vi "PCU_Connect.vi"(0 "GPIBBoard":i32, 1 "Address/ComPort":string, 2 "Communication":T1(ring), 3 "Terminator":enum32{"Cr", "Lf", "CrLf"}(ring), 4 "Portnumber":i32, 5 "error in":errorcluster, 6 "Target":enum32{"rdo100", "rdo110"}(radio), 7 "PCU-100 Control ID":string) -> (14 "Reference out":refnum<k24>, 19 "error out":errorcluster)   [LabVIEW 2017]
uses:
  C:/Users/Ssantec_Test/Documents/Instrument_DLL_Sample_Labview_20250826_Ver1.5.0_x64/DLL/InstrumentDLL.dll
  DLL/InstrumentDLL.dll
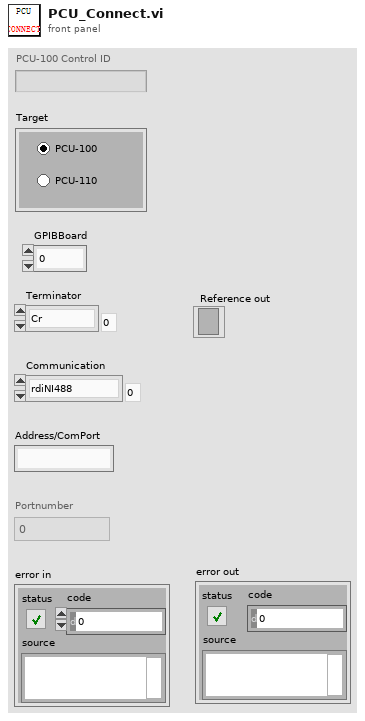
[diagram p1: front panel]
types:
  T1 = enum32{"rdiNI488", "rdiNIvisa", "rdikeysightvisa", "rdiUSB", "rdiLAN"}
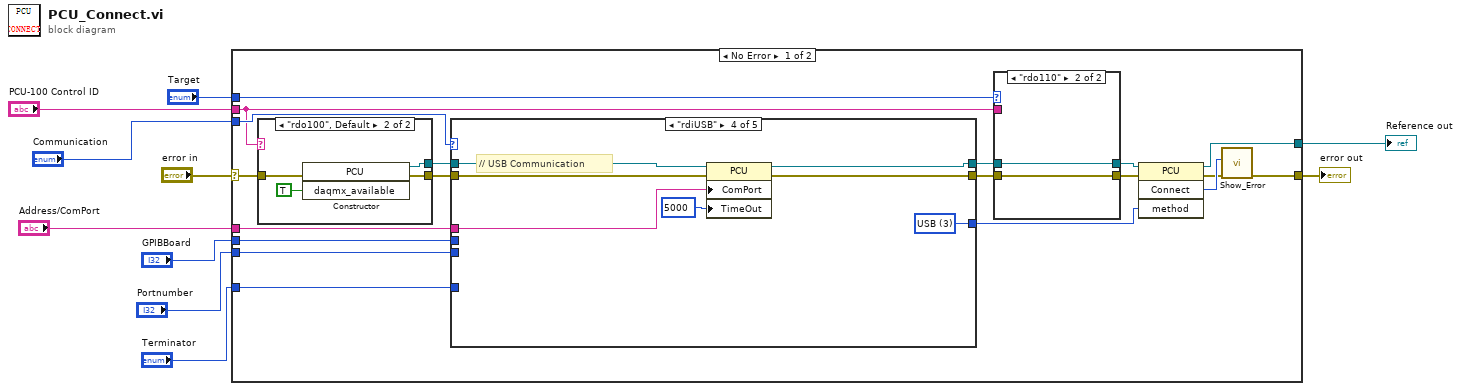
[diagram p0: block diagram]
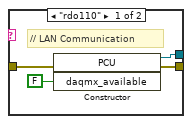
[diagram p2: hidden frame]
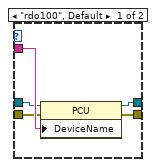
[diagram p3: hidden frame]
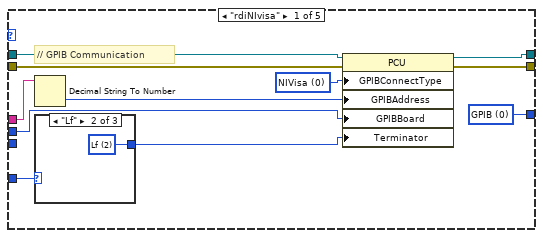
[diagram p4: hidden frame]
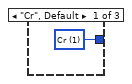
[diagram p5: hidden frame]
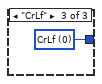
[diagram p6: hidden frame]
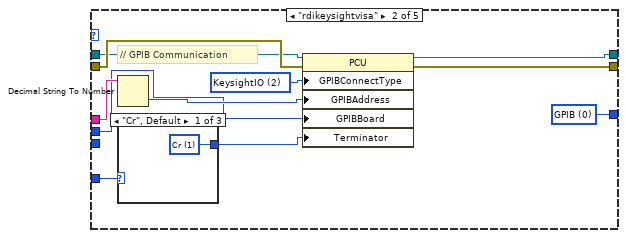
[diagram p7: hidden frame]
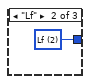
[diagram p8: hidden frame]
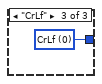
[diagram p9: hidden frame]
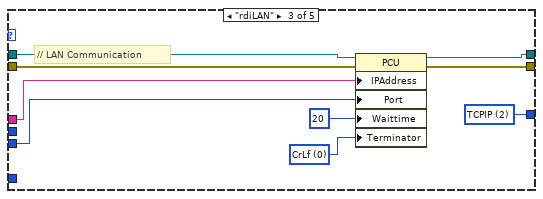
[diagram p10: hidden frame]
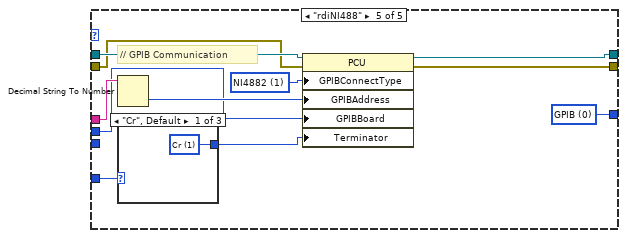
[diagram p11: hidden frame]
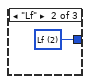
[diagram p12: hidden frame]
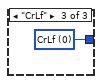
[diagram p13: hidden frame]
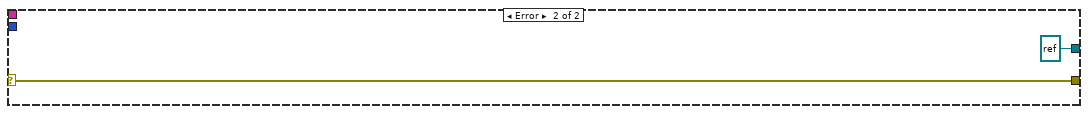
[diagram p14: hidden frame]
diagram:
  n1 = case shown="No Error" "error in" {
    selector: "error in" -> [w26 w104]
    tunnel: "Address/ComPort" -> [w29 _]
    tunnel: [w21 refnum<k24> refnum ("new reference")] -> w9
    tunnel: [w22 w104] -> w8
    tunnel: "Terminator" -> [w28 _]
    tunnel: "Communication" -> [w27 _]
    tunnel: "Portnumber" -> [w20 _]
    tunnel: "GPIBBoard" -> [w19 _]
    tunnel: "Target" -> [w18 _]
    tunnel: "PCU-100 Control ID" -> [w13 _]
    frame No Error {
      n2 = case shown="\"rdo100\", Default" w13 {
        tunnel: [w33 w37] -> w12
        tunnel: w26 -> [w32 w36]
        tunnel: [w31 w35] -> w11
        frame "rdo110" {
          # "// LAN Communication"
          n3 = constructor class="PCU"(error in=w32, "daqmx_available"=FALSE) -> (reference out=w33:refnum<k24>, error out=w31:errorcluster)  [unwired: 2 in, 2 out]
        }
        frame "rdo100", Default {
          n4 = constructor class="PCU"(error in=w36, "daqmx_available"=TRUE) -> (reference out=w37:refnum<k24>, error out=w35:errorcluster)  [unwired: 2 in, 2 out]
        }
      }
      n5 = case shown="\"rdiUSB\"" w27 {
        tunnel: w29 -> [w53 w67 w81 w87 w97]
        tunnel: w11 -> [w46 w60 w73 w83 w89]
        tunnel: w28 -> [w49 w63 _ _ w93]
        tunnel: [w50 w66 w77 w84 w94] -> w17
        tunnel: [w51 w65 w78 w85 w95] -> w16
        tunnel: [w52 w64 w79 w86 w96] -> w25
        tunnel: w20 -> [_ _ w75 _ _]
        tunnel: w19 -> [w47 w61 _ _ w91]
        tunnel: w12 -> [w45 w59 w74 w82 w90]
        frame "rdiNIvisa" {
          w52 = 0 items=["GPIB", "C232C", "TCPIP", "USB"] ("method")
          w55 = 0 items=["NIVisa", "NI4882", "KeysightIO"] ("GPIBConnectType")
          # "// GPIB Communication"
          n6 = Decimal String To Number(string=w53) -> (number=w54:i32)  [unwired: 2 in, 1 out]
          n7 = case shown="\"Lf\"" w49 {
            tunnel: [w56 w57 w58] -> w48
            frame "Cr", Default {
              w56 = 1 items=["CrLf", "Cr", "Lf"] ("Terminator")
            }
            frame "Lf" {
              w57 = 2 items=["CrLf", "Cr", "Lf"] ("Terminator")
            }
            frame "CrLf" {
              w58 = 0 items=["CrLf", "Cr", "Lf"] ("Terminator")
            }
          }
          n8 = property on="属性节点" class="PCU"(reference=w45, error in=w46, "GPIBConnectType"=w55, "GPIBAddress"=w54, "GPIBBoard"=w47, "Terminator"=w48) -> (reference out=w50:refnum<k24>, error out=w51:errorcluster)
        }
        frame "rdikeysightvisa" {
          w64 = 0 items=["GPIB", "C232C", "TCPIP", "USB"] ("method")
          w69 = 2 items=["NIVisa", "NI4882", "KeysightIO"] ("GPIBConnectType")
          # "// GPIB Communication"
          n9 = Decimal String To Number(string=w67) -> (number=w68:i32)  [unwired: 2 in, 1 out]
          n10 = case shown="\"Cr\", Default" w63 {
            tunnel: [w70 w71 w72] -> w62
            frame "Cr", Default {
              w70 = 1 items=["CrLf", "Cr", "Lf"] ("Terminator")
            }
            frame "Lf" {
              w71 = 2 items=["CrLf", "Cr", "Lf"] ("Terminator")
            }
            frame "CrLf" {
              w72 = 0 items=["CrLf", "Cr", "Lf"] ("Terminator")
            }
          }
          n11 = property on="属性节点" class="PCU"(reference=w59, error in=w60, "GPIBConnectType"=w69, "GPIBAddress"=w68, "GPIBBoard"=w61, "Terminator"=w62) -> (reference out=w66:refnum<k24>, error out=w65:errorcluster)
        }
        frame "rdiLAN" {
          w76 = 0 items=["CrLf", "Cr", "Lf"] ("Terminator")
          w79 = 2 items=["GPIB", "C232C", "TCPIP", "USB"] ("method")
          # "// LAN Communication"
          n12 = property on="属性节点" class="PCU"(reference=w74, error in=w73, "IPAddress"=w81, "Port"=w75, "Waittime"=20, "Terminator"=w76) -> (reference out=w77:refnum<k24>, error out=w78:errorcluster)
        }
        frame "rdiUSB" {
          w86 = 3 items=["GPIB", "C232C", "TCPIP", "USB"] ("method")
          # "// USB Communication"
          n13 = property on="属性节点" class="PCU"(reference=w82, error in=w83, "ComPort"=w87, "TimeOut"=5000 ("BaudRate")) -> (reference out=w84:refnum<k24>, error out=w85:errorcluster)
        }
        frame "rdiNI488" {
          w96 = 0 items=["GPIB", "C232C", "TCPIP", "USB"] ("method")
          w99 = 1 items=["NIVisa", "NI4882", "KeysightIO"] ("GPIBConnectType")
          # "// GPIB Communication"
          n14 = Decimal String To Number(string=w97) -> (number=w98:i32)  [unwired: 2 in, 1 out]
          n15 = case shown="\"Cr\", Default" w93 {
            tunnel: [w100 w101 w102] -> w92
            frame "Cr", Default {
              w100 = 1 items=["CrLf", "Cr", "Lf"] ("Terminator")
            }
            frame "Lf" {
              w101 = 2 items=["CrLf", "Cr", "Lf"] ("Terminator")
            }
            frame "CrLf" {
              w102 = 0 items=["CrLf", "Cr", "Lf"] ("Terminator")
            }
          }
          n16 = property on="属性节点" class="PCU"(reference=w90, error in=w89, "GPIBConnectType"=w99, "GPIBAddress"=w98, "GPIBBoard"=w91, "Terminator"=w92) -> (reference out=w94:refnum<k24>, error out=w95:errorcluster)
        }
      }
      n17 = case shown="\"rdo110\"" w18 {
        tunnel: w13 -> [w42 _]
        tunnel: w17 -> [w41 w44]
        tunnel: w16 -> [w40 w43]
        tunnel: [w39 w44] -> w15
        tunnel: [w38 w43] -> w14
        frame "rdo100", Default {
          n18 = property on="属性节点" class="PCU"(reference=w41, error in=w40, "DeviceName"=w42) -> (reference out=w39:refnum<k24>, error out=w38:errorcluster)
        }
        frame "rdo110" {
        }
      }
      n19 = invoke on="调用节点" class="PCU" method="Connect"(reference=w15, error in=w14, "method"=w25) -> (reference out=w21:refnum<k24>, error out=w23:errorcluster, "Connect"=w24:i32)  [unwired: 1 in, 1 out]
      n20 = call "Show_Error.vi"("error in (no error)"=w23, "Error"=w24) -> ("error out"=w22:errorcluster)  [unwired: 9 in]
    }
    frame Error {
    }
  }
  "Reference out" <- w9
  "error out" <- w8
